vi "PIO Write Read.vi"() -> ()   [LabVIEW 2016]
uses:
  Source/GE 5565PIORC/GE 5565PIORC Old.lvclass/GE 5565PIORC Old.ctl
  Source/GE 5565PIORC/VIs/Registers/Local Configuration.LAS1RR.Address Range.Get.vi
  Source/GE 5565PIORC/VIs/PIO/SubVIs/Byte Count to U32 Transfers.vi
  Source/GE 5565PIORC/VIs/PIO/SubVIs/PIO.Write U32 Array.vi
  Source/GE 5565PIORC/VIs/PIO/SubVIs/PIO.Write U8 Array.vi
  Source/GE 5565PIORC/VIs/PIO/SubVIs/PIO.Read U32 Array.vi
  Source/GE 5565PIORC/VIs/Registers/Local Configuration.Get Register Offset.vi
  Source/GE 5565PIORC/VIs/PIO/SubVIs/Change Endianness (1D U32).vi
  Source/GE 5565PIORC/VIs/PIO/SubVIs/Change Endianness (U32).vi
  Source/GE 5565PIORC/GE 5565PIORC Old.lvclass
panel:
  out "value":u8
  in  "offset":u32 format="%.0x"
  out "equal?":bool
  out "bytes read":u8[](array[numeric])
  in  "bytes to write":u8[](array[numeric])=[23, 255, 74, 2, 16, 17, 145, 67, 235, 160, 14]
  in  "VISA resource name":refnum<visa-resource-name>
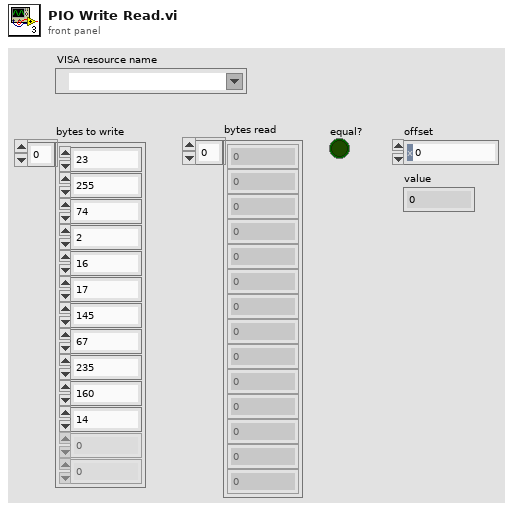
[diagram p1: front panel]
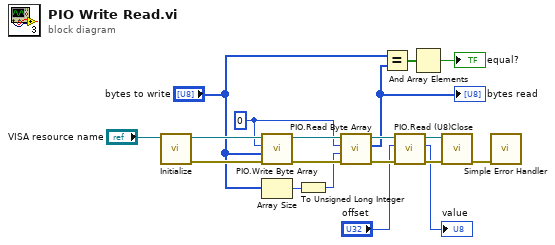
[diagram p0: block diagram]
diagram:
  w13 = u32 0 ("offset")
  n1 = call "Initialize.vi"("VISA resource name"="VISA resource name") -> ("error out"=w16:errorcluster, "GE 5565PIORC"=w17:refnum<class "GE 5565PIORC Old.lvclass">)  [unwired: 9 in]
  n2 = call "PIO.Write Byte Array.vi"("error in (no error)"=w16, "bytes to write"="bytes to write", "offset"=w13, "GE 5565PIORC in"=w17) -> ("error out"=w14:errorcluster, "GE 5565PIORC out"=w15:refnum<class "GE 5565PIORC Old.lvclass">)  [unwired: 6 in]
  n3 = Array Size(array="bytes to write") -> (size(s)=w10:i32)
  n4 = To Unsigned Long Integer(number=w10) -> (unsigned 32bit integer=w8:u32)
  n5 = call "PIO.Read Byte Array.vi"("error in (no error)"=w14, "count"=w8, "offset"=w13, "GE 5565PIORC in"=w15) -> ("error out"=w7:errorcluster, "bytes read"=w3:u8[], "GE 5565PIORC out"=w6:refnum<class "GE 5565PIORC Old.lvclass">)  [unwired: 5 in]
  "bytes read" <- w3
  n6 = Equal?(x="bytes to write", y=w3) -> (x = y?=w12:bool[])
  n7 = call "PIO.Read (U8).vi"("error in (no error)"=w7, "offset"="offset", "GE 5565PIORC in"=w6) -> ("error out"=w4:errorcluster, "value"=→"value":u8, "GE 5565PIORC out"=w5:refnum<class "GE 5565PIORC Old.lvclass">)  [unwired: 6 in]
  n8 = And Array Elements(Boolean array=w12) -> (logical AND=→"equal?":bool)
  n9 = call "Close.vi"("error in (no error)"=w4, "GE 5565PIORC in"=w5) -> ("error out"=w18:errorcluster)  [unwired: 8 in, 1 out]
  n10 = call <vilib>:"Simple Error Handler.vi"("error in (no error)"=w18) -> ()  [unwired: 4 in, 5 out]
